vi "UpdateSettings.channel.vi"(8 "error in (no error)":errorcluster, 11 "TektronixDPO in":refnum<class "TektronixDPO.lvclass">) -> (0 "error out":errorcluster, 3 "TektronixDPO out":refnum<class "TektronixDPO.lvclass">)   [LabVIEW 2013, in "TektronixDPO.lvclass"]
uses:
  TektronixDPO.lvclass
  shared/Typdefs/Choice78.ctl
  shared/Typdefs/Choice11.ctl
  shared/Typdefs/Choice79.ctl
  shared/OnOffTypeDef.ctl
  TektronixDPO.lvclass/TektronixDPO.ctl
  SupportClasses/TektronixDPOPhysicalDevice/TektronixDPO_PhysicalDevice.lvclass
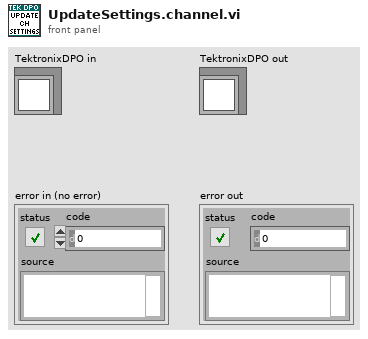
[diagram p1: front panel]
types:
  T1 = typedef "OnOffTypeDef.ctl" = enum16{"off", "on"}
  T2 = typedef "Choice79.ctl" = enum16{"FULL", "250 MHz", "150 MHz", "20 MHz"}
  T3 = typedef "Choice11.ctl" = enum16{"AC", "DC", "Ground"}
  T4 = typedef "Choice78.ctl" = enum16{"1M", "75", "50"}
  T5 = typedef "settings_TypDef.ctl" = cluster{"resourcename":string, "timeout":T6, "LocalSavingPath":path, "Save":T1, "Names":cluster{"Channel0":string, "Channel1":string, "Channel2":string, "Channel3":string, "Channel4":string}, "Calculations":T7, "NumChannels":T6, "NumMeasurements":T6, "NumPoints":T6, "waveformattributes":string, "Measurements":cluster{"Channel0":T6, "Channel1":T6, "Channel2":T6, "Channel3":T6}, "EnableMeasurements":T1, "Trigger":T13, "EnableReadWaveformInfo":T1, "probeattenuation":cluster{"Channel0":T6, "Channel1":T6, "Channel2":T6, "Channel3":T6}, "offset":cluster{"Channel0":T6, "Channel1":T6, "Channel2":T6, "Channel3":T6}, "Horizontal":T18, "verticalrange":cluster{"Channel0":T6, "Channel1":T6, "Channel2":T6, "Channel3":T6}, "Impedance":cluster{"Channel0":T4, "Channel1":T4, "Channel2":T4, "Channel3":T4}, "channelenabled":cluster{"Channel0":T1, "Channel1":T1, "Channel2":T1, "Channel3":T1}, "bandwidth":cluster{"Channel0":T2, "Channel1":T2, "Channel2":T2, "Channel3":T2}, "coupling":cluster{"Channel0":T3, "Channel1":T3, "Channel2":T3, "Channel3":T3}}
  T6 = typedef "BaseDriver.lvclass/numericVariable_TypeDef.ctl" = cluster{"Value":dbl, "Min":dbl, "Max":dbl, "StepSize":dbl, "Tolerance":dbl, "ValueActual":dbl}
  T7 = typedef "analysisTypDEf.ctl" = cluster{"Additional":T8, "Linked":T9, "Method":T11}
  T8 = typedef "additionalAnalysisCluster_TypDef.ctl" = cluster{"Analysis1":dbl, "Analysis2":dbl, "Analysis3":dbl, "Analysis4":dbl, "Analysis5":dbl, "Analysis6":dbl, "Analysis7":dbl, "Analysis8":dbl, "Analysis9":dbl, "Analysis10":dbl}
  T9 = typedef "LinkedChannelsCluster_TypDef.ctl" = cluster{"Analysis1":T10, "Analysis2":T10, "Analysis3":T10, "Analysis4":T10, "Analysis5":T10, "Analysis6":T10, "Analysis7":T10, "Analysis8":T10, "Analysis9":T10, "Analysis10":T10}
  T10 = typedef "channels_TypDef.ctl" = enum16{"Channel0", "Channel1", "Channel2", "Channel3", "Channel4", "Channel5", "Channel6", "Channel7", "n/a"}
  T11 = typedef "methodCluster_TypDEf.ctl" = cluster{"Analysis1":T12, "Analysis2":T12, "Analysis3":T12, "Analysis4":T12, "Analysis5":T12, "Analysis6":T12, "Analysis7":T12, "Analysis8":T12, "Analysis9":T12, "Analysis10":T12}
  T12 = typedef "method_TypDef.ctl" = enum16{"n/a", "max", "min", "energy", "trigger", "maxtime", "mintime"}
  T13 = typedef "TriggerCluster.ctl" = cluster{"Mode":T14, "Source":T15, "Coupling":T16, "Slope":T17, "Low Level":dbl}
  T14 = typedef "Choice73.ctl" = enum16{"Immediate", "Analog Edge"}
  T15 = typedef "Choice74.ctl" = enum16{"Channel 1", "Channel 2", "Channel 3", "Channel 4", "AC Line", "Aux", "Digital Channel 0", "Digital Channel 1", "Digital Channel 2", "Digital Channel 3", "Digital Channel 4", "Digital Channel 5", "Digital Channel 6", "Digital Channel 7", "Digital Channel 8", "Digital Channel 9", "Digital Channel 10", "Digital Channel 11", "Digital Channel 12", "Digital Channel 13", "Digital Channel 14", "Digital Channel 15", "RF"}
  T16 = typedef "Choice75.ctl" = enum16{"DC", "HF Reject", "LF Reject", "Noise Reject", "AC"}
  T17 = typedef "Choice76.ctl" = enum16{"Rising", "Falling"}
  T18 = typedef "Horizontal.ctl" = cluster{"time_window":dbl, "resolution":T19}
  T19 = typedef "Choice77.ctl" = enum16{"1E+3", "10E+3", "100E+3", "1E+6", "5E+6", "10E+6"}
  T20 = typedef "Choice78.ctl" = u16
  T21 = cluster{"Channel":T20, "offset":dbl, "verticalrange":dbl, "Impedance":u16, "Probe Attenuation":dbl, "Vertical Coupling":u16, "Bandwidth":u16, "Enabled":bool}
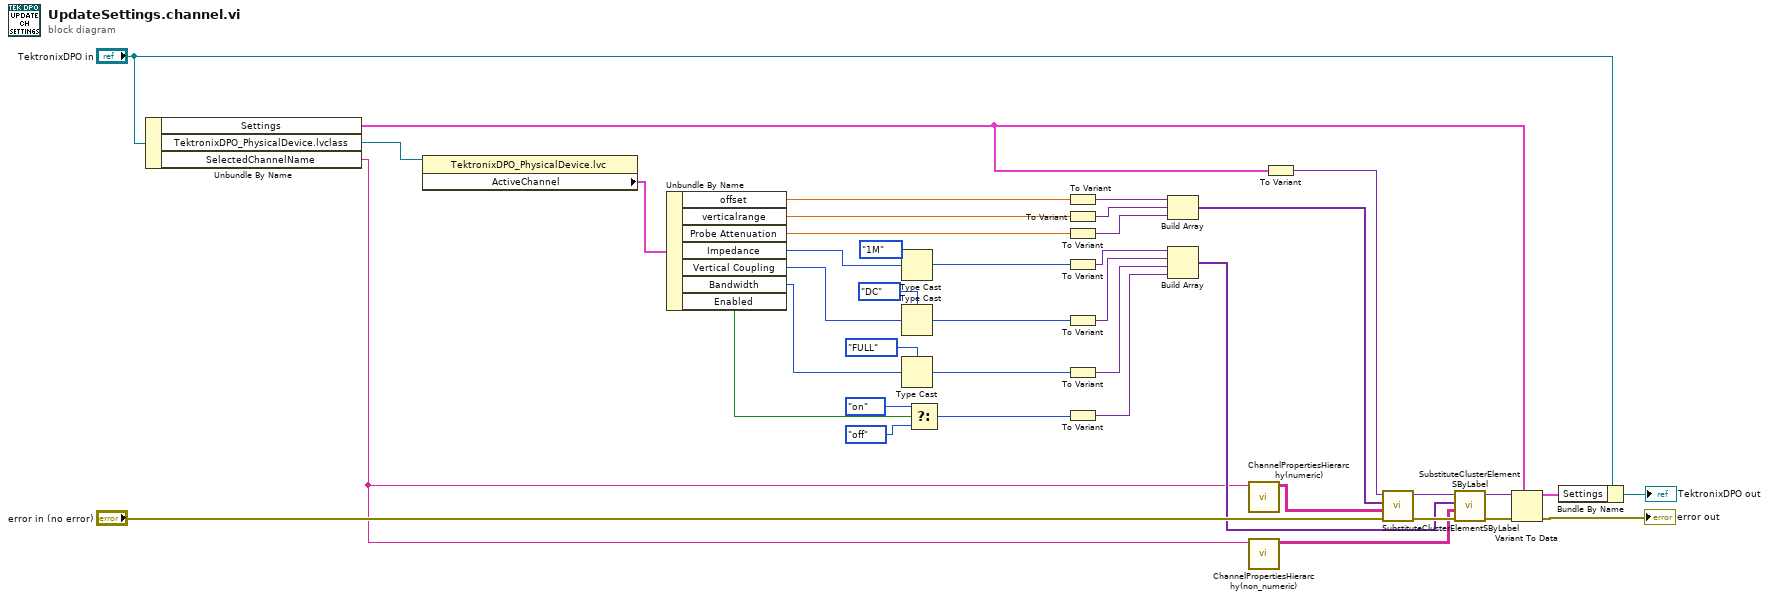
[diagram p0: block diagram]
diagram:
  n1 = Unbundle By Name("TektronixDPO in") -> ("Settings"=w27:T5, "TektronixDPO_PhysicalDevice.lvclass"=w37:refnum<class "TektronixDPO_PhysicalDevice.lvclass">, "SelectedChannelName"=w14:string)
  n2 = property class="TektronixDPO_PhysicalDevice.lvc"(reference=w37) -> ("ActiveChannel"=w35:T21)  [unwired: 1 in, 2 out]
  n3 = Unbundle By Name(w35) -> ("offset"=w34:dbl, "verticalrange"=w33:dbl, "Probe Attenuation"=w32:dbl, "Impedance"=w12:u16, "Vertical Coupling"=w10:u16, "Bandwidth"=w7:u16, "Enabled"=w4:bool)
  n4 = Type Cast(type=Choice78."1M" ("Impedance"), x=w12) -> (*(type *) &x=w11:T4)
  n5 = Type Cast(type=Choice11."DC" ("Vertical Coupling"), x=w10) -> (*(type *) &x=w8:T3)
  n6 = Type Cast(type=Choice79."FULL" ("Bandwidth"), x=w7) -> (*(type *) &x=w5:T2)
  n7 = Select(t=OnOffTypeDef."on" ("Channel0"), s=w4, f=OnOffTypeDef."off" ("Channel0")) -> (s? t:f=w1:T1)
  n8 = To Variant(anything=w34) -> (Variant=w31:variant)
  n9 = To Variant(anything=w33) -> (Variant=w30:variant)
  n10 = To Variant(anything=w32) -> (Variant=w29:variant)
  n11 = To Variant(anything=w11) -> (Variant=w26:variant)
  n12 = To Variant(anything=w8) -> (Variant=w25:variant)
  n13 = To Variant(anything=w5) -> (Variant=w24:variant)
  n14 = To Variant(anything=w1) -> (Variant=w23:variant)
  n15 = Build Array(w31, w30, w29) -> (w28:variant[])
  n16 = Build Array(w26, w25, w24, w23) -> (w16:variant[])
  n17 = call "ChannelPropertiesHierarchy(numeric).vi"("ChannelName"=w14) -> ("PropertiesHierarchy(numeric)"=w18:string[][])  [unwired: 10 in]
  n18 = call "ChannelPropertiesHierarchy(non_numeric).vi"("ChannelName"=w14) -> ("ElementsHierarchy"=w17:string[][])  [unwired: 10 in]
  n19 = To Variant(anything=w27) -> (Variant=w22:variant)
  n20 = call "SubstituteClusterElementSByLabel.vi"("error in (no error)"="error in (no error)", "ElementsHyerarchi"=w18, "NewElementsValues"=w28, "ClusterIn"=w22) -> ("error out"=w21:errorcluster, "UpdatedCluster out"=w20:variant)  [unwired: 6 in]
  n21 = call "SubstituteClusterElementSByLabel.vi"("error in (no error)"=w21, "ElementsHyerarchi"=w17, "NewElementsValues"=w16, "ClusterIn"=w20) -> ("error out"=w15:errorcluster, "UpdatedCluster out"=w19:variant)  [unwired: 6 in]
  n22 = Variant To Data(error in=w15, type=w27, Variant=w19) -> (data=w38:T5, error out=→"error out":errorcluster)
  n23 = Bundle By Name(cluster="TektronixDPO in", "Settings"=w38) -> (→"TektronixDPO out":refnum<class "TektronixDPO.lvclass">)
